vi "Brushed DC IO.vi"(6 "Brushed DC PWM Reverse":bool, 8 "Linear Amplifier Enable":bool, 9 "Brushed DC Motor Linear":sgl min=-100 max=100, 10 "Brushed DC Motor PWM":sgl min=-100 max=100, 11 "IO Cluster IN":T1) -> (0 "Error Out":errorcluster, 1 "Brushed DC Motor Filtered Current":sgl, 2 "Brushed DC Motor Speed (RPM)":dbl, 3 "IO Cluster OUT":T1)   [LabVIEW 2019]
uses:
  Actuators IO Cluster.ctl
  <vilib>/Utility/error.llb/Error Cluster From Error Code.vi
  <vilib>/rvi/errors/niLvFpgaAdjustHostInterfaceError.vi
  <vilib>/rvi/interface/nirviReadWriteControl/nirviReadWriteControl.xnode
  NiFpgaLv.dll
  <vilib>/rvi/interface/Simulation/niFpgaSimulationCallBeginRW.vi
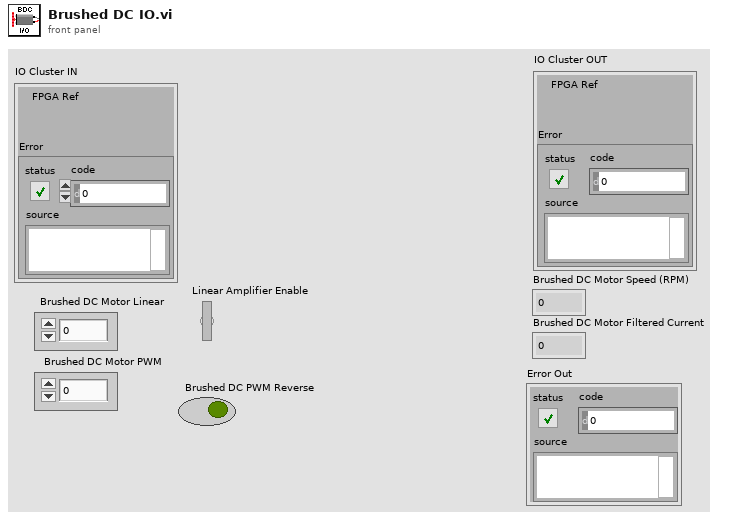
[diagram p1: front panel]
types:
  T1 = typedef "Actuators IO Cluster.ctl" = cluster{"Error":errorcluster, "FPGA Ref":refnum<k20>}
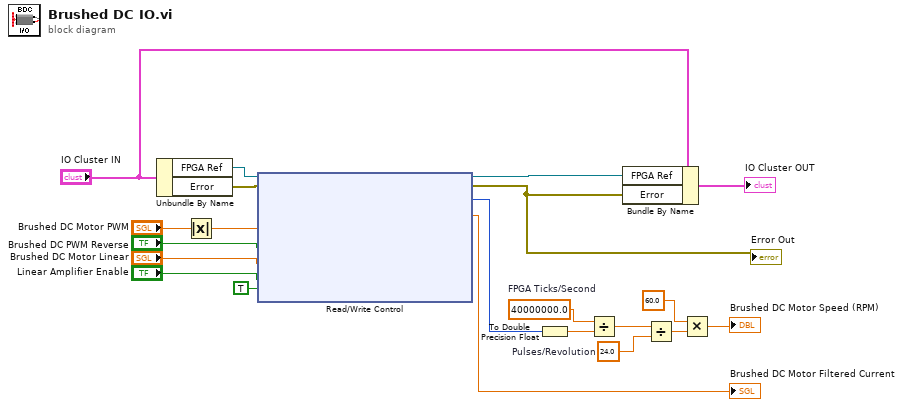
[diagram p0: block diagram]
diagram:
  w10 = 24.0  # Pulses/Revolution
  w18 = 40000000.0  # FPGA Ticks/Second
  n1 = Unbundle By Name("IO Cluster IN") -> ("FPGA Ref"=w7:refnum<k20>, "Error"=w6:errorcluster)
  n2 = Absolute Value(x="Brushed DC Motor PWM") -> (abs(x)=w1:sgl)
  n3 = xnode "Read/Write Control"("FPGA VI引用输入"=w7, "错误输入"=w6, "DC Motor PWM (0-1)"=w1, "DC Motor PWM Dir"="Brushed DC PWM Reverse", "DC Linear Amplifier Value (+/-10)"="Brushed DC Motor Linear", "DC Motor Linear Amplifier Enable"="Linear Amplifier Enable", "LED DC Motor"=TRUE) -> ("FPGA VI引用输出"=w14:refnum<k20>, "错误输出"=w13:errorcluster, "DC Motor Tach Ticks"=w20:u32, "DC Motor Filtered Current"=→"Brushed DC Motor Filtered Current":sgl)
  "Error Out" <- w13
  n4 = To Double Precision Float(number=w20) -> (double precision float=w19:dbl)
  n5 = Divide(x=w18, y=w19) -> (x/y=w11:dbl)
  n6 = Bundle By Name(cluster="IO Cluster IN", "FPGA Ref"=w14, "Error"=w13) -> (→"IO Cluster OUT":T1)
  n7 = Divide(x=w11, y=w10) -> (x/y=w9:dbl)
  n8 = Multiply(x=60.0, y=w9) -> (x*y=→"Brushed DC Motor Speed (RPM)":dbl)
